vi "DrawLinePlot.vi"(0 "reference in":refnum<class "LcWebView.lvclass">, 1 "XLabels":string[](array[string]), 2 "LinePlot.Dataset":dbl[](array[numeric]), 3 "LinePlot.DatasetLabels":string[](array[string]), 5 "Error In":errorcluster, 6 "GenericPlotOptions":T2, 7 "BarPlot.PlotColours":u32[](array[numeric]), 8 "BarPlotOptions":T1={"xLabel"="", "yLabel"="", "DisplayXLabel"=TRUE, "DisplayYLabel"=TRUE}) -> (14 "reference out":refnum<class "LcWebView.lvclass">, 19 "Error Out":errorcluster)   [LabVIEW 2018, in "LcWebView.lvclass"]
uses:
  LcWebView.lvclass
  ctrls/GenericPlotOption.ctl
  ctrls/LegendPosition.ctl
  ctrls/LinePlotOption.ctl
  cdfa7b6c-348e-4618-b79e-b8b55caa0d01.vi
  <vilib>/JDP Science/JSONtext/Variant to JSON Text.vi
  <vilib>/JDP Science/JSONtext/LVClass Serializer/JSONtext LVClass Serializer.lvclass
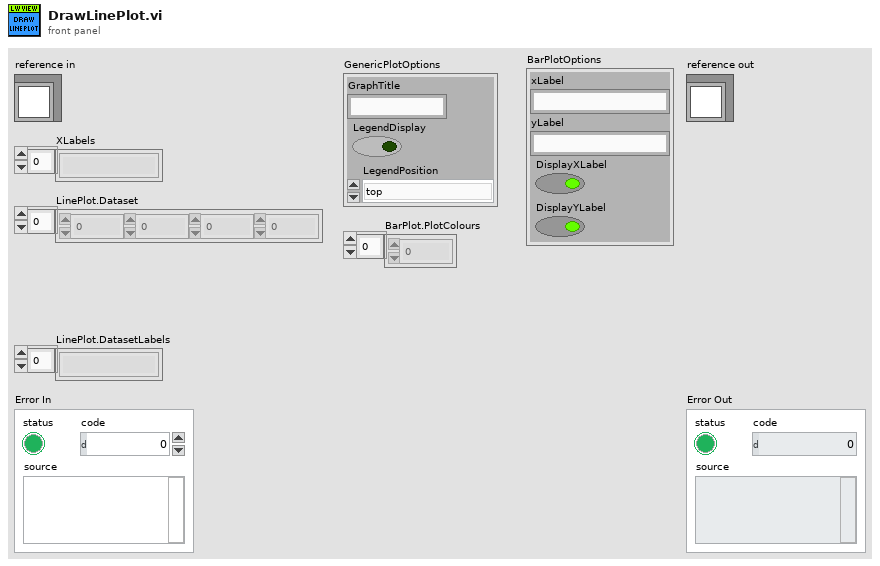
[diagram p1: front panel]
types:
  T1 = typedef "LcWebView.lvclass/LinePlotOption.ctl" = cluster{"xLabel":string, "yLabel":string, "DisplayXLabel":bool, "DisplayYLabel":bool}
  T2 = typedef "LcWebView.lvclass/GenericPlotOption.ctl" = cluster{"GraphTitle":string, "LegendDisplay":bool, "LegendPosition":T3}
  T3 = typedef "LcWebView.lvclass/LegendPosition.ctl" = enum16{"top", "right", "left", "bottom"}
  T4 = cluster{"action":string, "PlotData":string, "GenericPlotOptions":T2, "LinePlotOptions":T1}
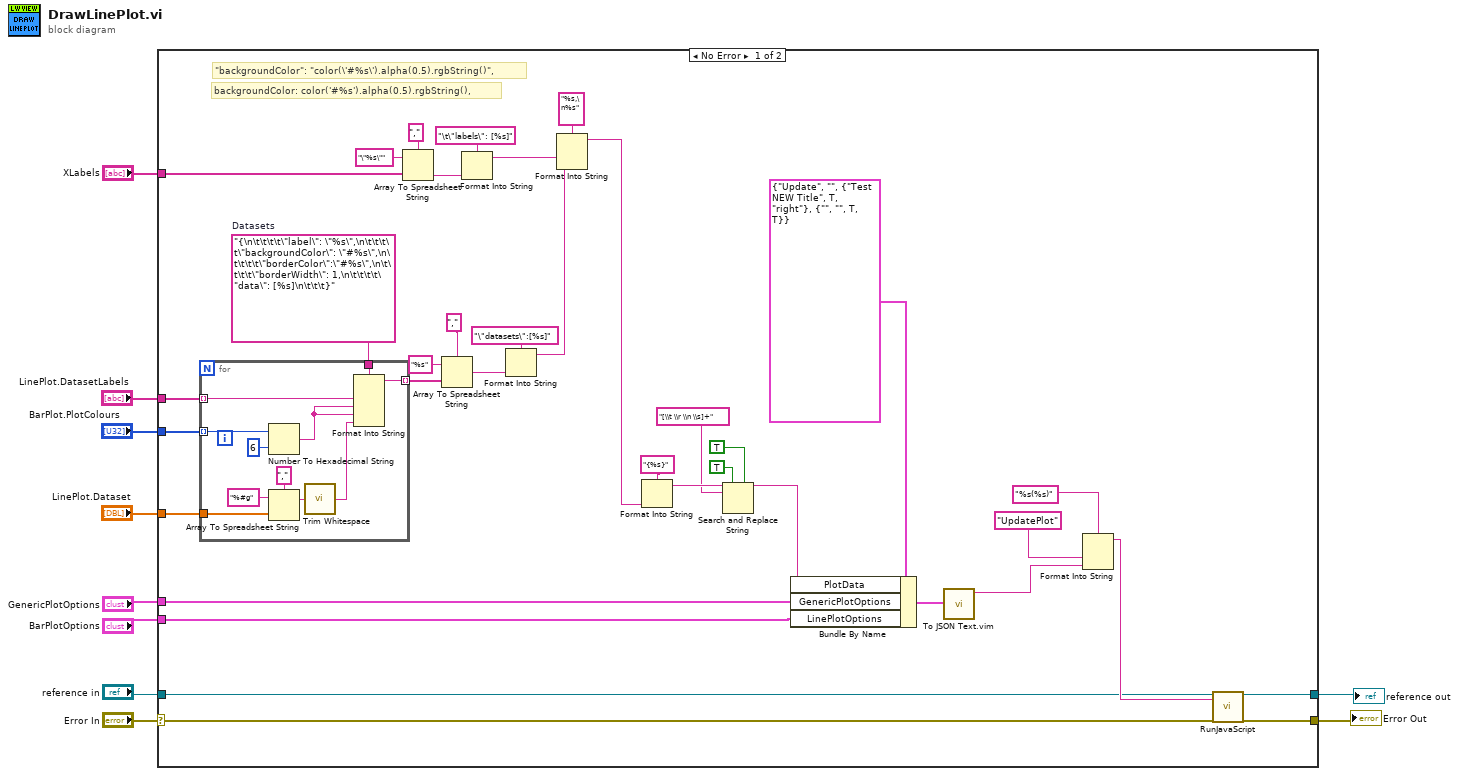
[diagram p0: block diagram]
diagram:
  n1 = case shown="No Error" "Error In" {
    selector: "Error In" -> [w15 w59]
    tunnel: [w16 w59] -> w1
    tunnel: [w17 w58] -> w2
    tunnel: "reference in" -> [w18 w58]
    tunnel: "LinePlot.Dataset" -> [w37 _]
    tunnel: "BarPlot.PlotColours" -> [w36 _]
    tunnel: "LinePlot.DatasetLabels" -> [w35 _]
    tunnel: "XLabels" -> [w34 _]
    tunnel: "GenericPlotOptions" -> [w26 _]
    tunnel: "BarPlotOptions" -> [w25 _]
    frame No Error {
      w38 = "{\n\t\t\t\t\"label\": \"%s\",\n\t\t\t\t\"backgroundColor\": \"#%s\",\n\t\t\t\t\"borderColor\":\"#%s\",\n\t\t\t\t\"borderWidth\": 1,\n\t\t\t\t\"data\": [%s]\n\t\t\t}"  # Datasets
      # "\"backgroundColor\": \"color(\\'#%s\\').alpha(0.5).rgbString()\","
      # "backgroundColor: color('#%s').alpha(0.5).rgbString(),"
      n2 = for {
        tunnel: w37 -> [w55]
        tunnel: w36 -> [w51] mode=indexing
        tunnel: w35 -> [w53] mode=indexing
        tunnel: [w52] -> w14 mode=indexing
        tunnel: w38 -> [w54]
        n3 = Number To Hexadecimal String(1:i16 6 ("width (-)"), 2:w51) -> (0:w50:string)
        n4 = Array To Spreadsheet String(delimiter (Tab)=",", array=w55, 3:"%#g" ("format string")) -> (spreadsheet string=w49:string)
        n5 = call <vilib>:"Trim Whitespace.vi"("string"=w49) -> ("trimmed string"=w48:string)  [unwired: 1 in]
        n6 = Format Into String(format string=w54, w53, w50, w50, w48) -> (resulting string=w52:string)  [unwired: 2 in, 1 out]
      }
      n7 = Array To Spreadsheet String(delimiter (Tab)=",", array=w34, 3:"\"%s\"" ("format string")) -> (spreadsheet string=w42:string)
      n8 = Array To Spreadsheet String(delimiter (Tab)="," ("separator"), array=w14, 3:"%s" ("format string")) -> (spreadsheet string=w11:string)
      n9 = Format Into String(format string="\t\"labels\": [%s]", w42) -> (resulting string=w45:string)  [unwired: 2 in, 1 out]
      n10 = Format Into String(format string="\"datasets\":[%s]", w11) -> (resulting string=w40:string)  [unwired: 2 in, 1 out]
      n11 = Format Into String(format string="%s,\n%s", w45, w40) -> (resulting string=w32:string)  [unwired: 2 in, 1 out]
      n12 = Format Into String(format string="{%s}", w32) -> (resulting string=w31:string)  [unwired: 2 in, 1 out]
      n13 = Search and Replace String(replace all?=TRUE ("replace all? (F)"), multiline?=TRUE ("multiline? (F)"), input string=w31, search string="[\\t \\r \\n \\s]+") -> (result string=w30:string)  [unwired: 4 in, 3 out]
      n14 = Bundle By Name(cluster=T4 {"action"="Update", "PlotData"="", "GenericPlotOptions"={"GraphTitle"="Test NEW Title", "LegendDisplay"=TRUE, "LegendPosition"=enum."right"}, "LinePlotOptions"={"xLabel"="", "yLabel"="", "DisplayXLabel"=TRUE, "DisplayYLabel"=TRUE}}, "PlotData"=w30, "GenericPlotOptions"=w26, "LinePlotOptions"=w25) -> (w23:T4)
      n15 = call "To JSON Text.vim"("Anything"=w23) -> ("<JSON>"=w20:string)  [unwired: 9 in, 1 out]
      n16 = Format Into String(format string="%s(%s)", "UpdatePlot" ("input 1"), w20) -> (resulting string=w19:string)  [unwired: 2 in, 1 out]
      n17 = call-dynamic "RunJavaScript.vi"("reference in"=w18, "Java Script Function"=w19, "Error In"=w15) -> ("reference out"=w17:refnum<class "LcWebView.lvclass">, "Error Out"=w16:errorcluster)  [unwired: 13 in, 2 out]
    }
    frame Error {
    }
  }
  "Error Out" <- w1
  "reference out" <- w2
